vi "save_spectra_h5.vi"(8 "error in (no error)":errorcluster, 9 "II channel seq IN":cluster{"BG":sgl[], "Ie":sgl[], "I0":sgl[]}[](array[cluster]), 10 "I channel seq IN":cluster{"BG":sgl[], "Ie":sgl[], "I0":sgl[]}[](array[cluster]), 11 "Detector in":refnum<class "Detector.lvclass">) -> (0 "error out":errorcluster, 3 "Detector out":refnum<class "Detector.lvclass">)   [LabVIEW 2020, in "Detector.lvclass"]
uses:
  Detector.lvclass
  <vilib>/addons/h5labview2/file/H5Fmode.ctl
  <vilib>/LabVIEW Open Source Project/Epoch Date & Time/epoch.UNIX/Epoch.UNIX.lvclass
  C:/Program Files (x86)/National Instruments/LabVIEW 2020/vi.lib/LabVIEW Open Source Project/Epoch Date & Time/epoch/Epoch.lvclass
  <vilib>/LabVIEW Open Source Project/Epoch Date & Time/Get Epoch Time.vi
  <vilib>/addons/h5labview2/file/H5F.lvlib
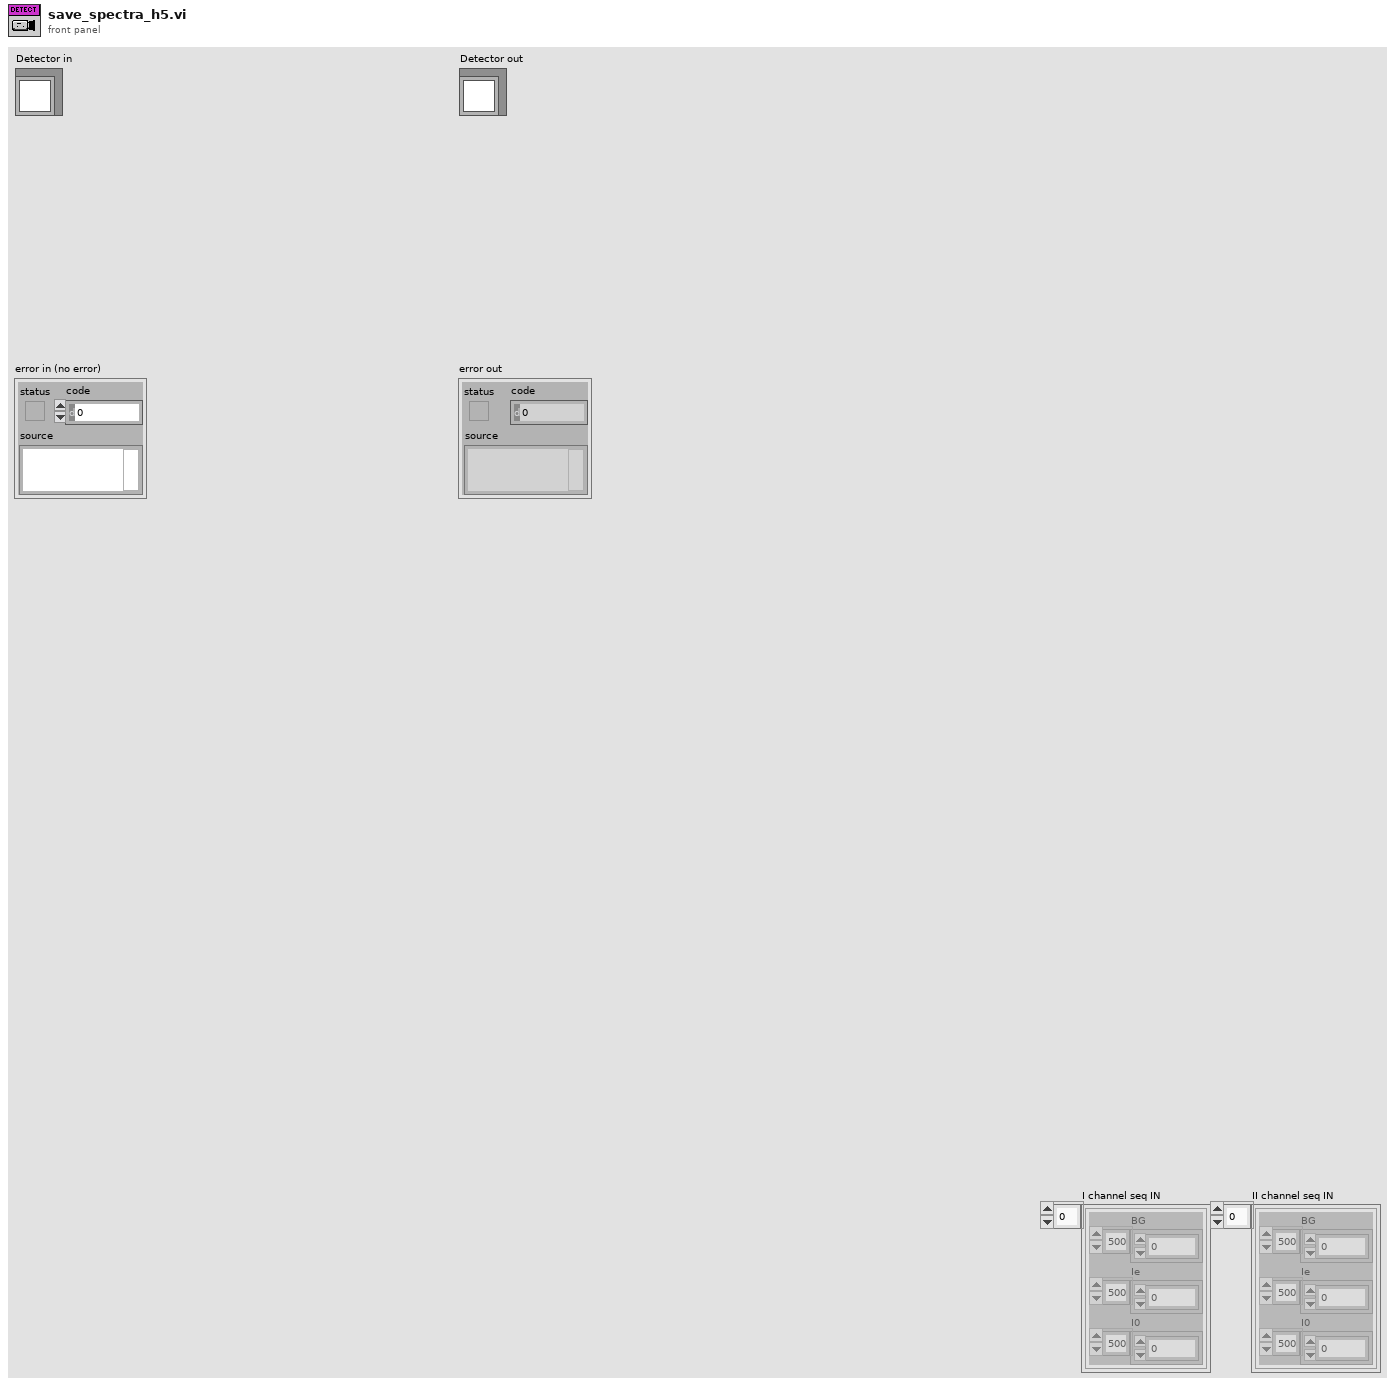
[diagram p1: front panel]
types:
  T1 = typedef "H5F.lvlib/H5Fmode.ctl" = enum16{"read-only", "read-write", "overwrite", "create new", "open or create"}
  T2 = typedef "hid_t.ctl" = i64
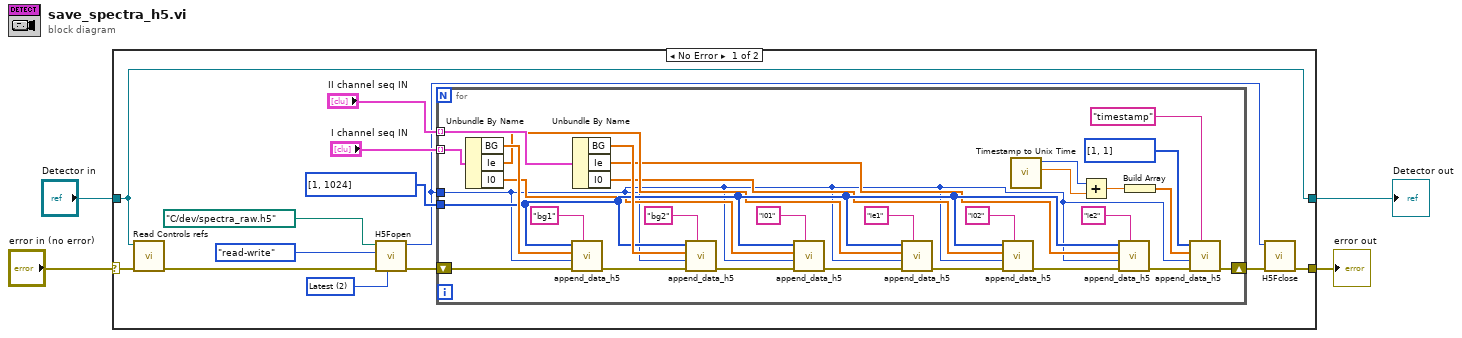
[diagram p0: block diagram]
diagram:
  n1 = case shown="No Error" "error in (no error)" {
    selector: "error in (no error)" -> [w16 w49]
    tunnel: [w5 w49] -> w3
    tunnel: [w17 w48] -> w1
    tunnel: "Detector in" -> [w17 w48]
    frame No Error {
      w10 = u16 2 items=["Earliest", "v1.8", "Latest"] ("compatibility")
      n2 = call "Read Controls refs.vi"("error in (no error)"=w16, "Detector in"=w17) -> ("error out"=w8:errorcluster)  [unwired: 7 in, 2 out]
      n3 = call <vilib>:"H5Fopen.vi"("compatibility"=w10, "error in (no error)"=w8, "mode (read-only)"=H5Fmode."read-write", "path"=path "C:/dev/spectra_raw.h5") -> ("error out"=w9:errorcluster, "ref out"=w6:T2)  [unwired: 6 in]
      n4 = for {
        tunnel: "I channel seq IN" -> [w47] mode=indexing
        tunnel: "II channel seq IN" -> [w46] mode=indexing
        tunnel: w6 -> [w19]
        tunnel: i16[] [1, 1024] ("initialized array") -> [w31]
        shift-right: [w23] -> w7
        shift-left: w9 -> [w42]
        n5 = Unbundle By Name(w47) -> ("BG"=w44:sgl[], "Ie"=w30:sgl[], "I0"=w29:sgl[])
        n6 = call "append_data_h5.vi"("name"="bg1", "error in (no error)"=w42, "ref h5_file"=w19, "data"=w44, "initialized array"=w31) -> ("error out"=w43:errorcluster)  [unwired: 6 in]
        n7 = Unbundle By Name(w46) -> ("BG"=w41:sgl[], "Ie"=w27:sgl[], "I0"=w28:sgl[])
        n8 = call "append_data_h5.vi"("name"="bg2", "error in (no error)"=w43, "ref h5_file"=w19, "data"=w41, "initialized array"=w31) -> ("error out"=w39:errorcluster)  [unwired: 6 in]
        n9 = call "append_data_h5.vi"("name"="i01", "error in (no error)"=w39, "ref h5_file"=w19, "data"=w29, "initialized array"=w31) -> ("error out"=w38:errorcluster)  [unwired: 6 in]
        n10 = call "append_data_h5.vi"("name"="ie1", "error in (no error)"=w38, "ref h5_file"=w19, "data"=w30, "initialized array"=w31) -> ("error out"=w37:errorcluster)  [unwired: 6 in]
        n11 = call "append_data_h5.vi"("name"="i02", "error in (no error)"=w37, "ref h5_file"=w19, "data"=w28, "initialized array"=w31) -> ("error out"=w36:errorcluster)  [unwired: 6 in]
        n12 = call <vilib>:"Timestamp to Unix Time.vi"() -> ("Fractional Second"=w25:dbl, "Unix Time (s)"=w26:i64)  [unwired: 10 in]
        n13 = Add(x=w26, y=w25) -> (x+y=w22:dbl)
        n14 = call "append_data_h5.vi"("name"="ie2", "error in (no error)"=w36, "ref h5_file"=w19, "data"=w27, "initialized array"=w31) -> ("error out"=w24:errorcluster)  [unwired: 6 in]
        n15 = Build Array(w22) -> (w21:dbl[])
        n16 = call "append_data_h5.vi"("name"="timestamp", "error in (no error)"=w24, "ref h5_file"=w19, "data"=w21, "initialized array"=i16[] [1, 1]) -> ("error out"=w23:errorcluster)  [unwired: 6 in]
      }
      n17 = call <vilib>:"H5Fclose.vi"("error in (no error)"=w7, "ref"=w6) -> ("error out"=w5:errorcluster)  [unwired: 9 in]
    }
    frame Error {
    }
  }
  "error out" <- w3
  "Detector out" <- w1
